vi "InitStackArray.vi"(8 "Fourth":refnum<class "ActionStack.lvclass">, 9 "Third":refnum<class "ActionStack.lvclass">, 10 "Second":refnum<class "ActionStack.lvclass">, 11 "First":refnum<class "ActionStack.lvclass">) -> (3 "Actions":refnum<class "ActionStack.lvclass">[](array[class]))   [LabVIEW 2024, in "ActionStack.lvclass"]
uses:
  ActionStack.lvclass
  ActionStack.lvclass/ActionStack.ctl
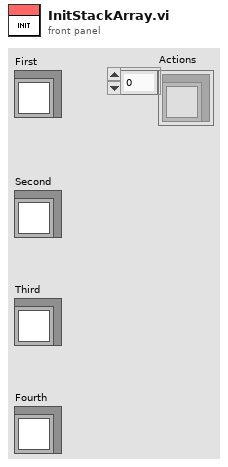
[diagram p1: front panel]
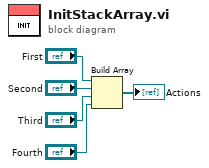
[diagram p0: block diagram]
diagram:
  n1 = Build Array("First", "Second", "Third", "Fourth") -> (→"Actions":refnum<class "ActionStack.lvclass">[])
